vi "Peak Density Find all Possible Neighbors.vi"(1 "Range (2)":i32=2, 2 "Upper Limits":T1, 3 "Point":T1) -> (0 "Possible Neighbor Points":T1[](array[typedef]))   [LabVIEW 2018, in "Video Cam Processor.lvclass"]
uses:
  Video Cam Processor.lvclass
  Private/Hull Point STYP.ctl
  17dac953-4a0a-4bbf-a026-f5420f49e0b7.vi
  17dac953-4a0a-4bbf-a026-f5420f49e0b7.vi/685fbcef-0ea3-4621-a3ec-8685b5c602df.vi
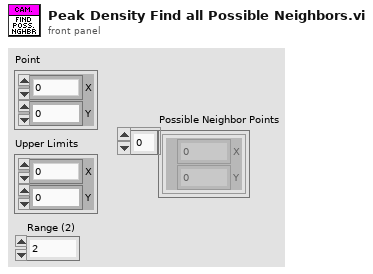
[diagram p1: front panel]
types:
  T1 = typedef "Video Cam Processor.lvclass/Hull Point STYP.ctl" = cluster{"X":i32, "Y":i32}
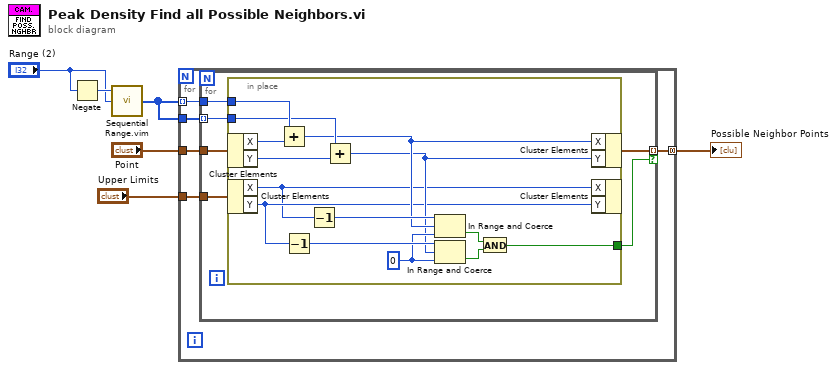
[diagram p0: block diagram]
diagram:
  n1 = Negate(x="Range (2)") -> (-x=w6:i32)
  n2 = call "Sequential Range.vim"("Stop (exc.)"="Range (2)", "Start (0, inc.)"=w6) -> ("Range(st, stp, inc)"=w4:i32[])  [unwired: 1 in]
  n3 = for {
    tunnel: w4 -> [w10] mode=indexing
    tunnel: w4 -> [w11]
    tunnel: "Point" -> [w9]
    tunnel: [w7] -> w1 mode=concatenating
    tunnel: "Upper Limits" -> [w8]
    n4 = for {
      tunnel: w11 -> [w15] mode=indexing
      tunnel: w10 -> [w16]
      tunnel: w9 -> [w17]
      tunnel: [w13] -> w7 mode=indexing if=w12
      tunnel: w8 -> [w14]
      n5 = in-place {
        in-place-border: w16 -> [w30]
        in-place-border: w15 -> [w28]
        in-place-border: [w18] -> w12
        w25 = 0
        n6 = in-place-cluster #1(w17) -> ("X"=w31:i32, "Y"=w29:i32)
        n7 = in-place-cluster #2(w14) -> ("X"=w21:i32, "Y"=w22:i32)
        n8 = Add(x=w30, y=w31) -> (x+y=w24:i32)
        n9 = Decrement(x=w22) -> (x-1=w26:i32)
        n10 = Decrement(x=w21) -> (x-1=w27:i32)
        n11 = Add(x=w28, y=w29) -> (x+y=w23:i32)
        n12 = In Range and Coerce(upper limit=w27, x=w24, lower limit=w25) -> (In Range?=w20:bool)  [unwired: 1 out]
        n13 = In Range and Coerce(upper limit=w26, x=w23, lower limit=w25) -> (In Range?=w19:bool)  [unwired: 1 out]
        n14 = And(x=w20, y=w19) -> (x .and. y?=w18:bool)
        n15 = in-place-cluster #1("X"=w24, "Y"=w23) -> (w13:T1)
        n16 = in-place-cluster #2("X"=w21, "Y"=w22) -> ()  [unwired: 1 out]
      }
    }
  }
  "Possible Neighbor Points" <- w1
